vi "NanotecSMCPD.set phase current.vi"(0 "i ref in":refnum<vi>, 1 "axis":i32, 2 "phase current [A]":dbl=1.0, 3 "ms timeout (10000)":i32=10000, 5 "error in (no error)":errorcluster) -> (14 "i ref out":refnum<vi>, 17 "timed out":bool, 19 "error out":errorcluster)   [LabVIEW 2014, in "NanotecSMCPD.lvlib"]
doc: "For the specified axis, sets the phase current."
uses:
  NanotecSMCPD.lvlib
  CSCore/CSSystem/CoreDefs/CoreDefs.error_type.ctl
  CSCore/CSSystem/CoreDefs/CoreDefs.error_severity.ctl
  CSCore/CSApplicationBaseClasses/DeviceBase/DeviceBase.lvlib
  CSCore/CSSystem/CoreLib/CoreLib.lvlib
  CSCore/CSApplicationBaseClasses/MotorBase/MotorBase.lvlib
  CSinstr.lib/NanotecSMCPD/NanotecSMCPDDriver.lvlib
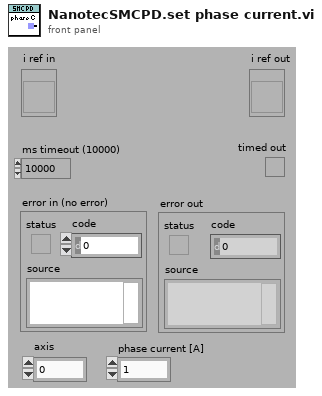
[diagram p1: front panel]
types:
  T1 = typedef "CoreDefs.error_severity.ctl" = enum16{"undefined", "information", "warning", "error", "fatal"}
  T2 = typedef "CoreDefs.error_type.ctl" = enum16{"no error", "can't load process", "can't unload process", "process does not exist", "can't install process", "can't remove process", "unknown function", "time out", "can't execute function", "duplicate queue name", "super not found", "caller queue invalid", "can't ping process", "unknown error", "VISA Error", "VISA timeout", "GPIB timeout", "GPIB error", "communication error", "data type mismatch", "can't read data from OPC server", "can't write data to OPC server", "OET error", "function not implemented", "process already exists", "invalid Shared Variable name", "error writing Shared Variable", "error reading Shared Variable", "invalid client name", "corrupt database", "unknown class", "call not authorized", "parameter out of range", "OET timeout: can't get data to modify", "invalid queue name", "requested operation incompatible with current state", "event undefined", "event disabled", "state undefined", "caller is not a friend", "EventBuilder: bad eventID", "EventBuilder: no DAQ devices", "a thread must not stop itself", "UNUSED ELEMENT4", "DiscArchiver: eventData incomplete", "DiscArchiver: eventData does not belong to run", "DiscArchiver: can't open file", "DiscArchiver: can't write to file", "DiscArchiver: available disc space low", "can't acquire semaphore", "error reading data from database", "notifier object is not existing", "can't register process", "can't unregister process", "illegal event type", "object disabled", "object already exists", "can't change state", "Instrument not found", "no connection to remote node", "invalid reference", "N/A", "UNUSED ELEMENT 1", "element not found", "illegal TCP/IP connection detected", "object does not exist", "invalid access ID", "unknown CS system", "invalid privilige", "unsupported data type", "unsupported server type", "IO server already exists", "Shared Variable already exists"}
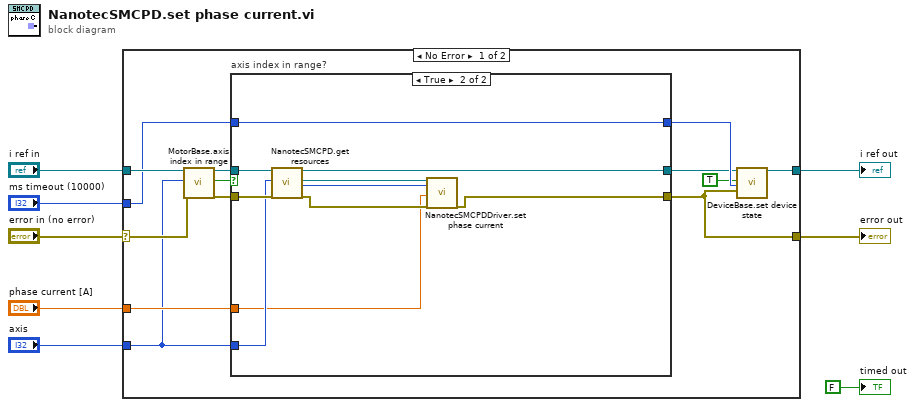
[diagram p0: block diagram]
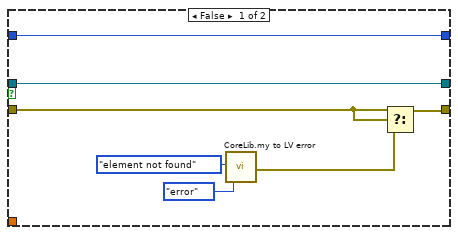
[diagram p2: hidden frame]
diagram:
  n1 = case shown="No Error" "error in (no error)" {
    selector: "error in (no error)" -> [w14 w39]
    tunnel: "ms timeout (10000)" -> [w10 _]
    tunnel: "i ref in" -> [w15 w40]
    tunnel: [w13 w39] -> w5
    tunnel: "axis" -> [w11 _]
    tunnel: [w9 w40] -> w3
    tunnel: "phase current [A]" -> [w12 _]
    frame No Error {
      n2 = call "MotorBase.axis index in range.vi"("i ref in"=w15, "axisIndex"=w11, "error in (no error)"=w14) -> ("i ref out"=w19:refnum<vi>, "in range"=w18:bool, "error out"=w20:errorcluster)  [unwired: 14 in]
      n3 = case "axis index in range?" shown="True" w18 {
        tunnel: [w28 w31] -> w17
        tunnel: [w25 w30] -> w13
        tunnel: w10 -> [w22 w38]
        tunnel: w12 -> [_ w29]
        tunnel: w11 -> [_ w35]
        tunnel: w19 -> [w28 w36]
        tunnel: w20 -> [w26 w37]
        tunnel: [w22 w38] -> w21
        frame False {
          n4 = call "CoreLib.my to LV error.vi"("ErrorTypes"=CoreDefs.error_type."element not found", "severityLevel"=CoreDefs.error_severity."error") -> ("myErrorCluster"=w24:errorcluster)  [unwired: 16 in, 1 out]
          n5 = Select(t=w26, s=w26, f=w24) -> (s? t:f=w25:errorcluster)
        }
        frame True {
          n6 = call "NanotecSMCPD.get resources.vi"("i ref in"=w36, "axisNumber"=w35, "error in (no error)"=w37) -> ("i ref out"=w31:refnum<vi>, "VISA resource"=w34:refnum<visa-resource-name>, "address"=w32:i32, "error out"=w33:errorcluster)  [unwired: 13 in]
          n7 = call "NanotecSMCPDDriver.set phase current.vi"("VISA resource name"=w34, "contollerID"=w32, "phaseCurrent [A]"=w29, "error in (no error)"=w33) -> ("error out"=w30:errorcluster)  [unwired: 13 in, 2 out]
        }
      }
      n8 = call "DeviceBase.set device state.vi"("i ref in"=w17, "implicit"=TRUE, "ms timeout (10000)"=w21, "device error"=w13) -> ("i ref out"=w9:refnum<vi>)  [unwired: 13 in, 2 out]
    }
    frame Error {
    }
  }
  "error out" <- w5
  "i ref out" <- w3
  "timed out" <- FALSE ("timed out")
